vi "Current Elevator State.vi"(8 "error in (no error)":errorcluster, 10 "Elevator State":T1 {"Current Elevation" scale=0.0..100.0; "Current Travel Rate" scale=-1.0..1.0}, 11 "GTH-Up in":refnum<class "GTH-Up.lvclass">) -> (0 "error out":errorcluster, 3 "GTH-Up out":refnum<class "GTH-Up.lvclass">)   [LabVIEW 2014, in "Elevator.lvlib" / "EL-Go To Height.lvlib" / "GTH-Up.lvclass"]
uses:
  GTH-Up.lvclass
  Elevator Class/Elevator State.ctl
  <vilib>/ActorFramework/Actor/Actor.lvclass/Actor.ctl
  <vilib>/ActorFramework/Message Enqueuer/Message Enqueuer.lvclass/Message Enqueuer.ctl
  <vilib>/ActorFramework/Message Enqueuer/Init from Existing Queue.vi
  <vilib>/ActorFramework/Message Enqueuer/Enqueue.vi
  <vilib>/ActorFramework/Message Priority Queue/Priority Enqueue.vi
  <vilib>/ActorFramework/Message Enqueuer/Message Enqueuer.lvclass
  EL-Go To Height Messages/Go To Holding Msg/Go To Holding Msg.lvclass
  EL-Go To Height Class/EL-Go To Height.lvclass
  <vilib>/ActorFramework/Actor/Actor.lvclass
  Elevator Class/Elevator.lvclass
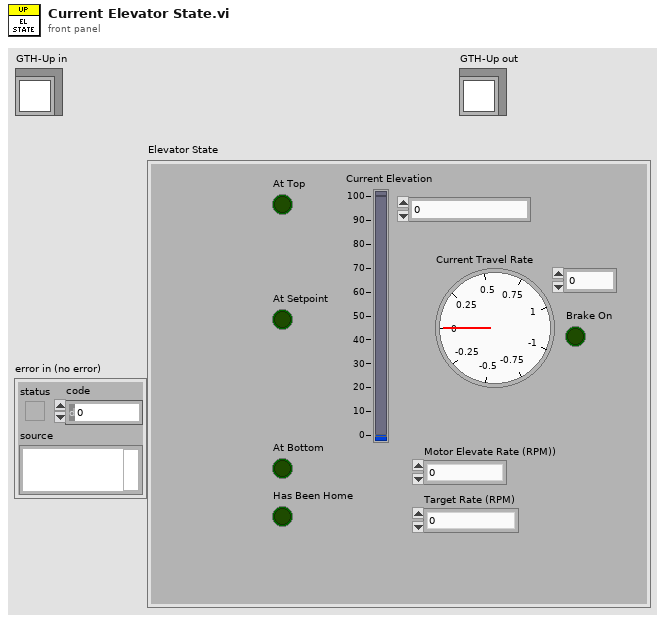
[diagram p1: front panel]
types:
  T1 = typedef "Elevator.lvlib/Elevator.lvclass/Elevator State.ctl" = cluster{"At Bottom":bool, "At Top":bool, "At Setpoint":bool, "Target Rate (RPM)":dbl, "Current Travel Rate":dbl, "Current Elevation":dbl, "Brake On":bool, "Motor Elevate Rate (RPM))":dbl, "Has Been Home":bool}
  T2 = typedef "Elevator.lvlib/EL-Go To Height.lvlib/EL-Go To Height.lvclass/Parameters.ctl" = cluster{"Target Height":dbl, "Elevator State Loop (ms)":u32, "Up Rate (Percentage)":dbl, "Down Rate (Percentage)":dbl}
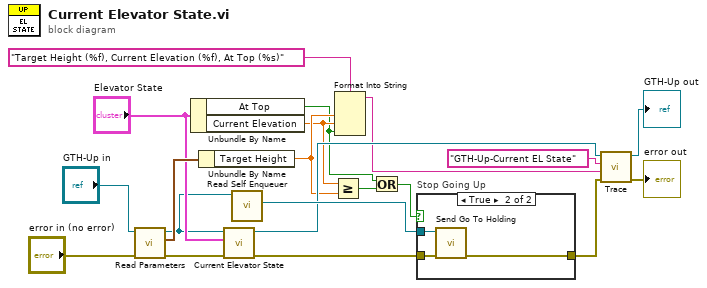
[diagram p0: block diagram]
diagram:
  n1 = call-dynamic "Read Parameters.vi"("error in (no error)"="error in (no error)", "EL-Go To Height in"="GTH-Up in") -> ("error out"=w3:errorcluster, "Parameters"=w19:T2, "EL-Go To Height out"=w15:refnum<class "GTH-Up.lvclass">)  [unwired: 7 in]
  n2 = Unbundle By Name("Elevator State") -> ("At Top"=w6:bool, "Current Elevation"=w7:dbl)
  n3 = Unbundle By Name(w19) -> ("Target Height"=w8:dbl)
  n4 = call-parent "Current Elevator State.vi"("error in (no error)"=w3, "Elevator State"="Elevator State", "EL-Go To Height in"=w15) -> ("error out"=w2:errorcluster, "EL-Go To Height out"=w13:refnum<class "GTH-Up.lvclass">)  [unwired: 7 in]
  n5 = call <vilib>:"Read Self Enqueuer.vi"("Actor"=w15) -> ("Self Enqueuer"=w14:refnum<class "Message Enqueuer.lvclass">)  [unwired: 10 in]
  n6 = Greater Or Equal?(x=w7, y=w8) -> (x >= y?=w16:bool)
  n7 = Format Into String(format string="Target Height (%f), Current Elevation (%f), At Top (%s)", w8, w7, w6) -> (resulting string=w5:string)  [unwired: 2 in, 1 out]
  n8 = Or(x=w6, y=w16) -> (x .or. y?=w17:bool)
  n9 = case "Stop Going Up" shown="True" w17 {
    tunnel: w14 -> [_ w24]
    tunnel: w2 -> [w21 w23]
    tunnel: [w21 w22] -> w1
    frame False {
    }
    frame True {
      n10 = call "Send Go To Holding.vi"("error in (no error)"=w23, "Message Enqueuer"=w24) -> ("error out"=w22:errorcluster)  [unwired: 8 in, 1 out]
    }
  }
  n11 = call-dynamic "Trace.vi"("error in (no error)"=w1, "Command Message"=w5, "Command Action"="GTH-Up-Current EL State", "Command Actor in"=w13) -> ("error out"=→"error out":errorcluster, "Command Actor out"=→"GTH-Up out":refnum<class "GTH-Up.lvclass">)  [unwired: 6 in]
